vi "疫苗簇数组转字符串数组.vi"(1 "疫苗信息":T1[](array[typedef]) {"生产日期" format="%<%Y/%m/%d>T"}) -> (0 "疫苗信息":string[][](table))   [LabVIEW 2018]
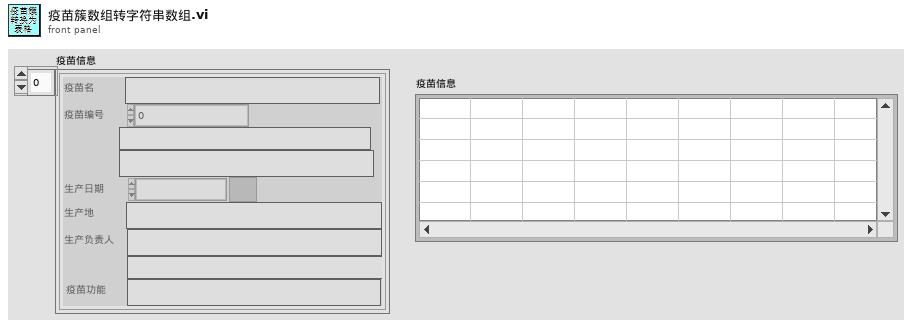
[diagram p1: front panel]
types:
  T1 = typedef "疫苗信息.ctl" = cluster{"疫苗名":string, "疫苗编号":i32, "疫苗类型":string, "生产厂家":string, "生产日期":timestamp, "生产地":string, "生产负责人":string, "是否合格":string, "疫苗功能":string}
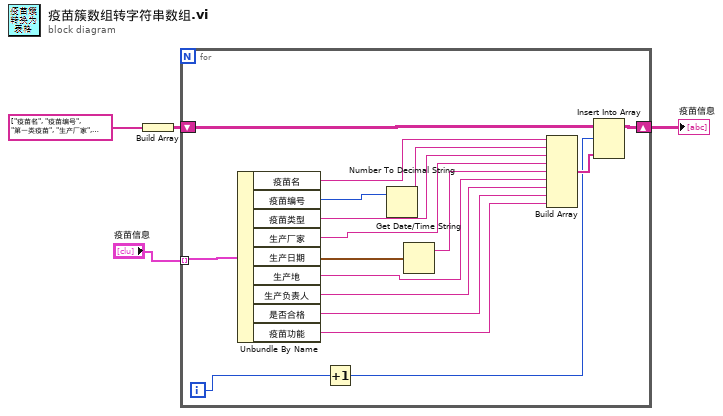
[diagram p0: block diagram]
diagram:
  n1 = Build Array(string[] ["疫苗名", "疫苗编号", "第一类疫苗", "生产厂家", "生产日期", "生产地", "生产负责人", "检验合格", "疫苗功能"] ("columns")) -> (w3:string[][])
  n2 = for {
    tunnel: "疫苗信息" -> [w21] mode=indexing
    shift-right: [w9] -> w1
    shift-left: w3 -> [w10]
    i -> [w8]
    n3 = Unbundle By Name(w21) -> ("疫苗名"=w19:string, "疫苗编号"=w20:i32, "疫苗类型"=w6:string, "生产厂家"=w13:string, "生产日期"=w17:timestamp, "生产地"=w15:string, "生产负责人"=w14:string, "是否合格"=w5:string, "疫苗功能"=w12:string)
    n4 = Increment(x=w8) -> (x+1=w7:i32)
    n5 = Number To Decimal String(number=w20) -> (decimal integer string=w18:string)  [unwired: 1 in]
    n6 = Get Date/Time String(seconds (now)=w17) -> (date string=w16:string)  [unwired: 2 in, 1 out]
    n7 = Build Array(w19, w18, w6, w13, w16, w15, w14, w5, w12) -> (w11:string[])
    n8 = Insert Into Array(array=w10, index (row)=w7, new element=w11) -> (w9:string[][])  [unwired: 1 in]
  }
  "疫苗信息" <- w1
